vi "DecodeSignedThousandths.vi"(1 "Data In":u8[](array[numeric])) -> (0 "Data Out":dbl[](array[numeric]))   [LabVIEW 2015, in "navX Library v1 (deprecated).lvlib"]
uses:
  navX Library v1 (deprecated).lvlib
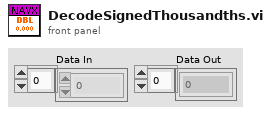
[diagram p1: front panel]
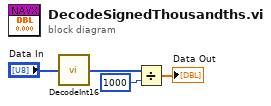
[diagram p0: block diagram]
diagram:
  n1 = call "DecodeInt16.vi"("Data In"="Data In") -> ("Data Out"=w1:i16[])
  n2 = Divide(x=w1, y=1000) -> (x/y=→"Data Out":dbl[])
